vi "List Group Objects (recursive).vi"(6 "error in (no error)":errorcluster, 7 "Object Types (any)":T1[](array[typedef]) items=["H5G_UNKNOWN"=-1, "H5G_GROUP"=0, "H5G_DATASET"=1, "H5G_TYPE"=2, "H5G_LINK"=3, "H5G_UDLINK"=4], 8 "pattern":string, 9 "HDF5 Loc Ref":T2) -> (0 "error out":errorcluster, 1 "Object Types":T1[](array[typedef]) items=["H5G_UNKNOWN"=-1, "H5G_GROUP"=0, "H5G_DATASET"=1, "H5G_TYPE"=2, "H5G_LINK"=3, "H5G_UDLINK"=4], 2 "Object Names":string[](array[string]), 3 "HDF5 Loc Ref out":T2)   [LabVIEW 2017]
doc: "Lists some or all of the objects at a given location"
uses:
  <vilib>/UPVI/lvhdf5/group.llb/H5G_obj_t.ctl
  <vilib>/UPVI/lvhdf5/library.llb/HDF5 Ref.ctl
  <userlib>/_OpenG.lib/array/array.llb/Conditional Auto-Indexing Tunnel (I32)__ogtk.vi
  <userlib>/_OpenG.lib/array/array.llb/Conditional Auto-Indexing Tunnel (String)__ogtk.vi
panel:
  # "LVHDF5 Toolkit\nCopyright (c) 2005-2013 by Jason D. Sommerville\nCopyright (c) 2014 by UPVI, LLC.\n\nThis use and distribution of this file is governed by the terms found in \nLICENSE.txt distributed with this toolkit and installed at\n <user.lib>\\_lvhdf5\\LICENSE.txt"
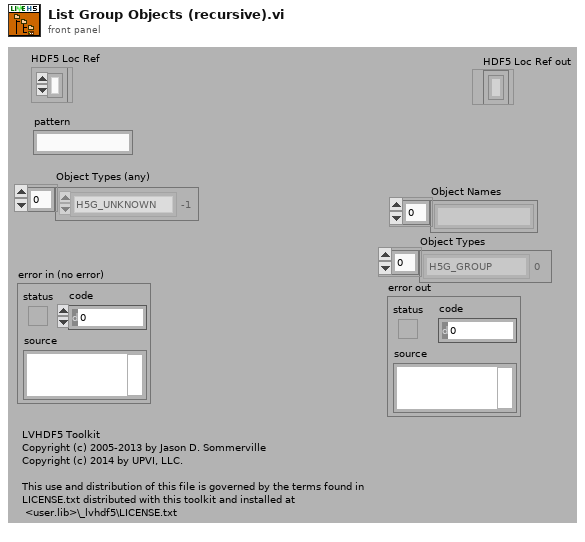
[diagram p1: front panel]
types:
  T1 = typedef "H5G_obj_t.ctl" = i32
  T2 = typedef "HDF5 Ref.ctl" = refnum<k1>
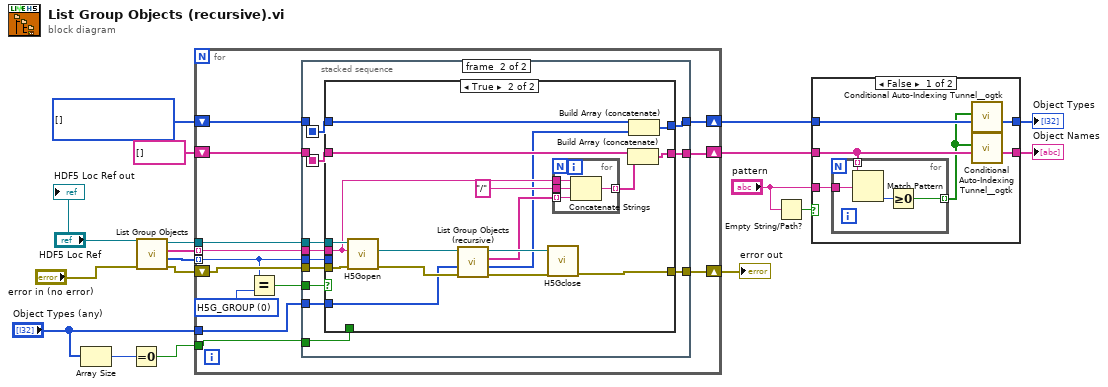
[diagram p0: block diagram]
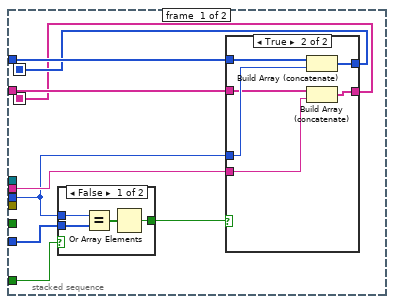
[diagram p3: hidden frame]
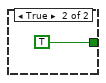
[diagram p5: hidden frame]
diagram:
  w13 = T1[] [] items=["H5G_UNKNOWN"=-1, "H5G_GROUP"=0, "H5G_DATASET"=1, "H5G_TYPE"=2, "H5G_LINK"=3, "H5G_UDLINK"=4]
  n1 = Array Size(array="Object Types (any)") -> (size(s)=w4:i32)
  n2 = Equal To 0?(x=w4) -> (x = 0?=w3:bool)
  n3 = call <vilib>:"List Group Objects.vi"("error in (no error)"="error in (no error)", "HDF5 Loc Ref"="HDF5 Loc Ref") -> ("error out"=w17:errorcluster, "Obect Types"=w16:T1[], "Object Names"=w18:string[], "HDF5 Loc Ref out"=w15:T2)  [unwired: 4 in]
  n4 = for {
    tunnel: w18 -> [w27] mode=indexing
    shift-right: [w20] -> w10
    shift-left: w17 -> [w31]
    tunnel: w16 -> [w24] mode=indexing
    tunnel: w15 -> [w30]
    shift-right: [w29] -> w9
    shift-left: string[] [] -> [w28]
    tunnel: "Object Types (any)" -> [w25]
    tunnel: w3 -> [w23]
    shift-right: [w22] -> w8
    shift-left: w13 -> [w21]
    w19 = T1 0 items=["H5G_UNKNOWN"=-1, "H5G_GROUP"=0, "H5G_DATASET"=1, "H5G_TYPE"=2, "H5G_LINK"=3, "H5G_UDLINK"=4] ("Object Type")
    n5 = Equal?(x=w24, y=w19) -> (x = y?=w26:bool)
    n6 = stacked-sequence {
      seq-local: [w34 _] -> [_ w55]
      seq-local: [w33 _] -> [_ w54]
      tunnel: w31 -> [_ w65]
      tunnel: w30 -> [_ w64]
      tunnel: [_ w63] -> w29
      tunnel: w28 -> [w39 _]
      tunnel: w27 -> [w38 w62]
      tunnel: w26 -> [_ w61]
      tunnel: w25 -> [w36 w60]
      tunnel: w24 -> [w37 w59]
      tunnel: w23 -> [w35 w58]
      tunnel: [_ w57] -> w22
      tunnel: w21 -> [w40 _]
      tunnel: [_ w56] -> w20
      frame #0 {
        n7 = case shown="False" w35 {
          tunnel: w36 -> [w52 _]
          tunnel: w37 -> [w51 _]
          tunnel: [w49 TRUE] -> w32
          frame False {
            n8 = Equal?(x=w51, y=w52) -> (x = y?=w50:bool[])
            n9 = Or Array Elements(Boolean array=w50) -> (logical OR=w49:bool)
          }
          frame True {
          }
        }
        n10 = case shown="True" w32 {
          tunnel: w39 -> [w41 w43]
          tunnel: [w42 w48] -> w34
          tunnel: w40 -> [w42 w47]
          tunnel: w37 -> [_ w46]
          tunnel: w38 -> [_ w45]
          tunnel: [w41 w44] -> w33
          frame False {
          }
          frame True {
            n11 = Build Array (concatenate)(w47, w46) -> (w48:T1[])
            n12 = Build Array (concatenate)(w43, w45) -> (w44:string[])
          }
        }
      }
      frame #1 {
        n13 = case shown="True" w61 {
          tunnel: w65 -> [w66 w85]
          tunnel: w64 -> [_ w84]
          tunnel: [w67 w83] -> w63
          tunnel: w54 -> [w67 w82]
          tunnel: w62 -> [_ w77]
          tunnel: w60 -> [_ w72]
          tunnel: w59 -> [_ _]
          tunnel: w58 -> [_ _]
          tunnel: [w68 w80] -> w57
          tunnel: w55 -> [w68 w81]
          tunnel: [w66 w76] -> w56
          frame False {
          }
          frame True {
            n14 = call <vilib>:"H5Gopen.vi"("error in (no error)"=w85, "Name"=w77, "HDF5 Ref"=w84) -> ("error out"=w73:errorcluster, "HDF5 Group Ref"=w75:T2)  [unwired: 4 in, 1 out]
            n15 = call <vilib>:"List Group Objects (recursive).vi"("error in (no error)"=w73, "Object Types (any)"=w72, "HDF5 Loc Ref"=w75) -> ("error out"=w69:errorcluster, "Object Types"=w70:T1[], "Object Names"=w71:string[], "HDF5 Loc Ref out"=w74:T2)  [unwired: 3 in]
            n16 = call <vilib>:"H5Gclose.vi"("error in (no error)"=w69, "HDF5 Group Ref"=w74) -> ("error out"=w76:errorcluster)  [unwired: 7 in]
            n17 = for {
              tunnel: w77 -> [w89]
              tunnel: w71 -> [w88] mode=indexing
              tunnel: "/" -> [w87]
              tunnel: [w86] -> w78 mode=indexing
              n18 = Concatenate Strings(w89, w87, w88) -> (w86:string)
            }
            n19 = Build Array (concatenate)(w82, w78) -> (w83:string[])
            n20 = Build Array (concatenate)(w81, w70) -> (w80:T1[])
          }
        }
      }
    }
  }
  "error out" <- w10
  n21 = Empty String/Path?(string/path="pattern") -> (empty?=w5:bool)
  n22 = case shown="False" w5 {
    tunnel: "pattern" -> [w95 _]
    tunnel: w9 -> [w94 w100]
    tunnel: w8 -> [w93 w101]
    tunnel: [w91 w101] -> w7
    tunnel: [w90 w100] -> w6
    frame False {
      n23 = for {
        tunnel: w95 -> [w99]
        tunnel: [w97] -> w92 mode=indexing
        tunnel: w94 -> [w96] mode=indexing
        n24 = Match Pattern(string=w96, regular expression=w99) -> (offset past match=w98:i32)  [unwired: 1 in, 3 out]
        n25 = Greater Or Equal To 0?(x=w98) -> (x >= 0?=w97:bool)
      }
      n26 = call-poly <userlib>:"Conditional Auto-Indexing Tunnel__ogtk.vi"("Array in"=w93, "Elements to keep"=w92) -> ("Filtered Array out"=w91:i32[])  [unwired: 5 in]
      n27 = call-poly <userlib>:"Conditional Auto-Indexing Tunnel__ogtk.vi"("Array in"=w94, "Elements to keep"=w92) -> ("Filtered Array out"=w90:string[])  [unwired: 5 in]
    }
    frame True {
    }
  }
  "Object Names" <- w6
  "Object Types" <- w7
  "HDF5 Loc Ref out" <- "HDF5 Loc Ref"
